vi "StartButtonPress.vi"(8 "error in (no error)":errorcluster, 11 "View in":refnum<class "View.lvclass">) -> (0 "error out":errorcluster, 3 "View out":refnum<class "View.lvclass">)   [LabVIEW 2024, in "GUI.lvlib" / "View.lvclass"]
uses:
  View.lvclass
  View.lvclass/View.ctl
  Controller/Controller.lvclass
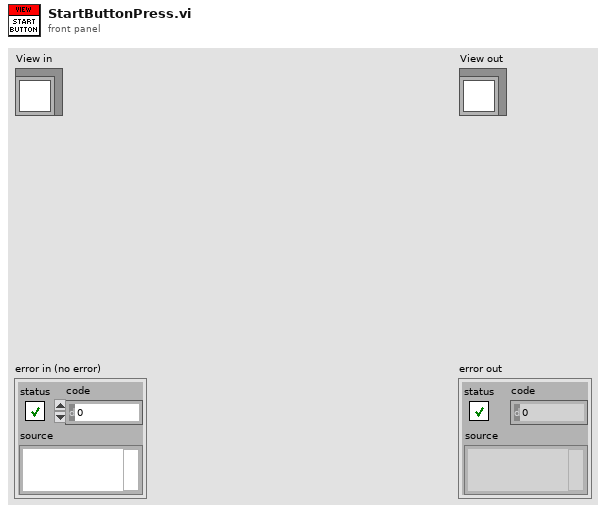
[diagram p1: front panel]
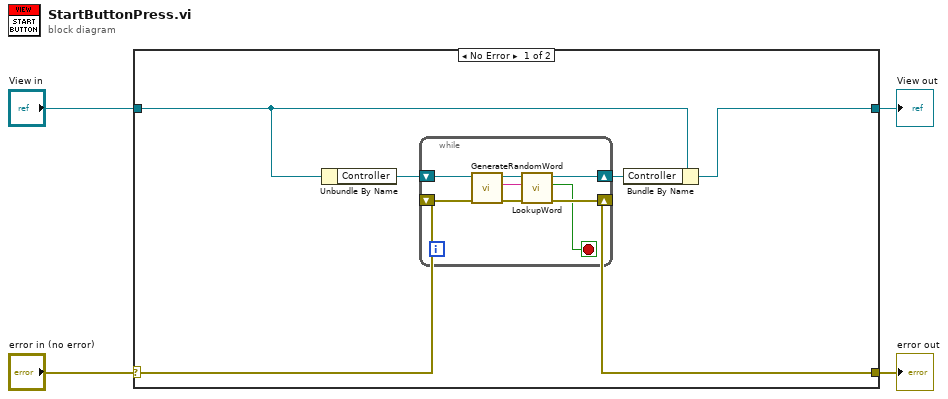
[diagram p0: block diagram]
diagram:
  n1 = case shown="No Error" "error in (no error)" {
    selector: "error in (no error)" -> [w6 w19]
    tunnel: [w5 w19] -> w3
    tunnel: [w7 w18] -> w1
    tunnel: "View in" -> [w9 w18]
    frame No Error {
      n2 = Unbundle By Name(w9) -> ("Controller"=w10:refnum<class "Controller.lvclass">)
      n3 = while {
        shift-right: [w16] -> w8
        shift-left: w10 -> [w17]
        shift-right: [w12] -> w5
        shift-left: w6 -> [w15]
        stop <- w11 stop-if-true
        n4 = call "GenerateRandomWord.vi"("Controller in"=w17, "error in (no error)"=w15) -> ("Controller out"=w16:refnum<class "Controller.lvclass">, "Word"=w14:string, "error out"=w13:errorcluster)  [unwired: 6 in]
        n5 = call "LookupWord.vi"("error in (no error)"=w13, "Word"=w14) -> ("error out"=w12:errorcluster, "Exists?"=w11:bool)  [unwired: 7 in, 1 out]
      }
      n6 = Bundle By Name(cluster=w9, "Controller"=w8) -> (w7:refnum<class "View.lvclass">)
    }
    frame Error {
    }
  }
  "error out" <- w3
  "View out" <- w1
